vi "HoloLink_link.vi"(8 "error in (no error)":errorcluster, 9 "memory":i32, 10 "searchRange":T1, 11 "session in":refnum<k35>) -> (0 "error out":errorcluster, 2 "FeaturesLinked":dbl[][](array[numeric]), 3 "Refnum out":refnum<k35>)   [LabVIEW 2023, in "holoTracker.lvlib"]
uses:
  holoTracker.lvlib
panel:
  # "wavelenght, optical_index, image_size_X, image_size_Y, pixel_size, magnification = holo_info\n\n    propag_param, focus_param, binarisation_param, CCL_param = analyse_parameters\n    distance_ini, nb_plane, propag_step, filter = propag_param\n    high_pass_filter, low_pass_filter = filter\n    #focus parameters unpacking\n    focus_type, sum_size = focus_param\n    #binarisation parameters unpacking\n    nbStdVarThreshold, threshold_target = binarisation_param\n    #CCL parameters unpacking\n    n_connectivity, min_voxel, max_voxel = CCL_param"
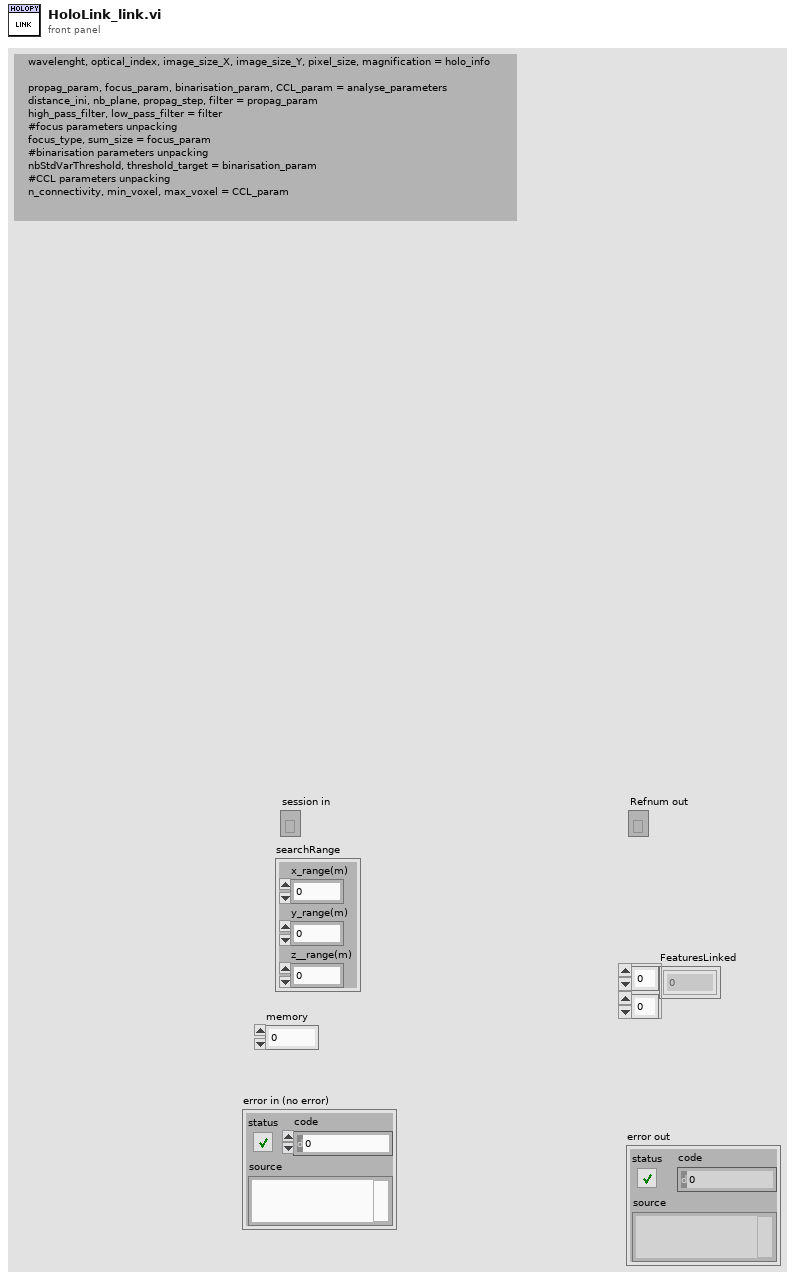
[diagram p1: front panel]
types:
  T1 = cluster{"x_range(m)":dbl, "y_range(m)":dbl, "z__range(m)":dbl}
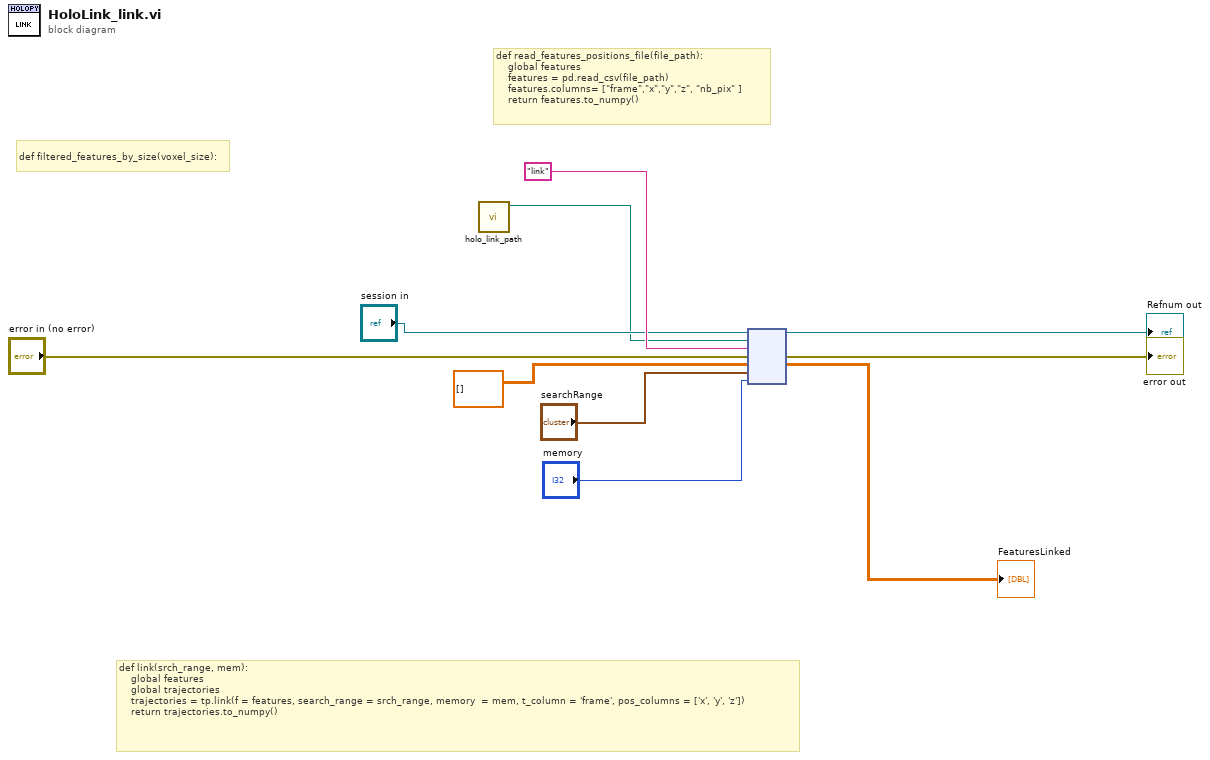
[diagram p0: block diagram]
diagram:
  # "def link(srch_range, mem):\n    global features\n    global trajectories\n    trajectories = tp.link(f = features, search_range = srch_range, memory  = mem, t_column = 'frame', pos_columns = ['x', 'y', 'z'])\n    return trajectories.to_numpy()"
  # "def filtered_features_by_size(voxel_size):"
  # "def read_features_positions_file(file_path):\n    global features\n    features = pd.read_csv(file_path)\n    features.columns= [\"frame\",\"x\",\"y\",\"z\", \"nb_pix\" ]\n    return features.to_numpy()"
  n1 = call "holo_link_path.vi"() -> ("appended path"=w7:path)  [unwired: 11 in]
  n2 = node("session in", w7, "link" ("function name"), "error in (no error)", dbl[][] [] ("FeaturesLinked"), "searchRange", "memory") -> (→"Refnum out":refnum<k35>, →"error out":errorcluster, →"FeaturesLinked":dbl[][])  [unwired: 2 in, 2 out]
